vi "ROE200_VisaRead.vi"(8 "error in (no error)":errorcluster, 10 "Expected Bytes":u32, 11 "Visa Reference In":refnum<visa-resource-name>) -> (0 "error out":errorcluster, 1 "return count":u32, 2 "read buffer":string, 3 "VISA resource  out":refnum<visa-resource-name>)   [LabVIEW 2019]
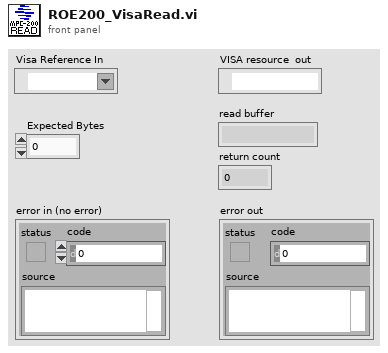
[diagram p1: front panel]
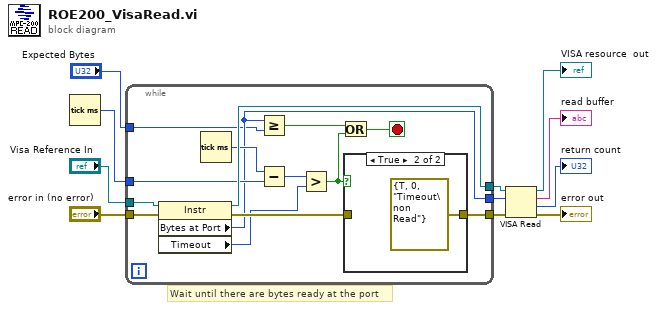
[diagram p0: block diagram]
diagram:
  # "Wait until there are bytes ready at the port"
  n1 = Tick Count (ms)() -> (millisecond timer value=w2:u32)
  n2 = while {
    tunnel: "Visa Reference In" -> [w25]
    tunnel: [w20] -> w10
    tunnel: [w24] -> w9
    tunnel: [w14] -> w8
    tunnel: "error in (no error)" -> [w22]
    tunnel: w2 -> [w17]
    tunnel: "Expected Bytes" -> [w13]
    stop <- w23 stop-if-true
    n3 = property class="Instr"(reference=w25, error in=w22) -> (reference out=w24:refnum<visa-resource-name>, error out=w19:errorcluster, "Bytes at Port"=w14:u32, "Timeout"=w12:u32)
    n4 = Tick Count (ms)() -> (millisecond timer value=w18:u32)
    n5 = Greater Or Equal?(x=w14, y=w13) -> (x >= y?=w15:bool)
    n6 = Subtract(x=w18, y=w17) -> (x-y=w16:u32)
    n7 = Greater?(x=w16, y=w12) -> (0:w21:bool)
    n8 = Or(x=w15, y=w21) -> (x .or. y?=w23:bool)
    n9 = case shown="True" w21 {
      tunnel: [w26 errorcluster {"status"=TRUE, "code"=0, "source"="Timeout\non Read"} ("error constant")] -> w20
      tunnel: w19 -> [w26 _]
      frame False {
      }
      frame True {
      }
    }
  }
  n10 = VISA Read(VISA resource name=w9, byte count=w8, error in (no error)=w10) -> (VISA resource name out=→"VISA resource  out":refnum<visa-resource-name>, read buffer=→"read buffer":string, return count=→"return count":u32, error out=→"error out":errorcluster)
